vi "getReadStatus.vi"(8 "error in (no error)":errorcluster, 11 "IReaderStatus in":refnum<class "IReaderStatus.lvclass">) -> (0 "error out":errorcluster, 2 "ReadStatus":T1 items=["Ok"=0, "Event"=1, "Fail"=2, "Unknown"=65535], 3 "IReaderStatus out":refnum<class "IReaderStatus.lvclass">)   [LabVIEW 2022 SP3, in "openDAQ.lvlib" / "IBaseObject.lvlib" / "IReaderStatus.lvlib" / "IReaderStatus.lvclass"]
uses:
  <instrlib>/openDAQ/Public/Classes/IReaderStatus/IReaderStatus.lvclass
  C:/Program Files (x86)/National Instruments/LabVIEW 2022/instr.lib/openDAQ/Public/Classes/IBaseObject/IBaseObject.lvclass
  <instrlib>/openDAQ/Public/TypeDef/ReadStatus.ctl
  <instrlib>/openDAQ/Public/Classes/IBaseObject/IBaseObject.lvclass/IBaseObject.ctl
  <instrlib>/openDAQ/Public/Classes/IBaseObject/Accessor/Read reference.vi
  <instrlib>/openDAQ/Public/Classes/IBaseObject/Accessor/Write reference.vi
  <instrlib>/openDAQ/Binaries/Windows/x86/copendaq32.dll
  <instrlib>/openDAQ/openDAQ.lvlib
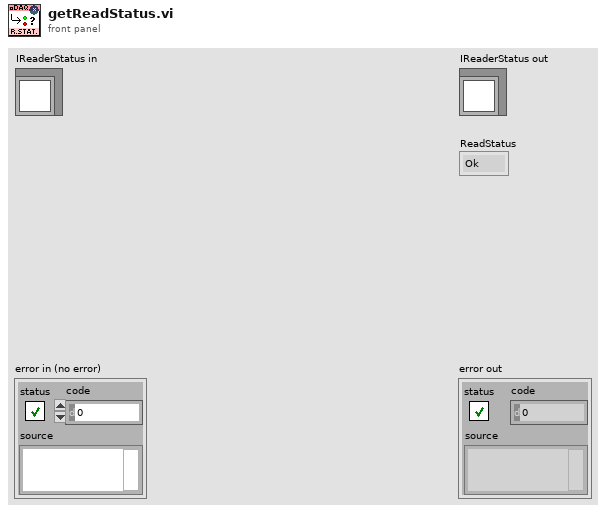
[diagram p1: front panel]
types:
  T1 = typedef "openDAQ.lvlib/ReadStatus.ctl" = u16
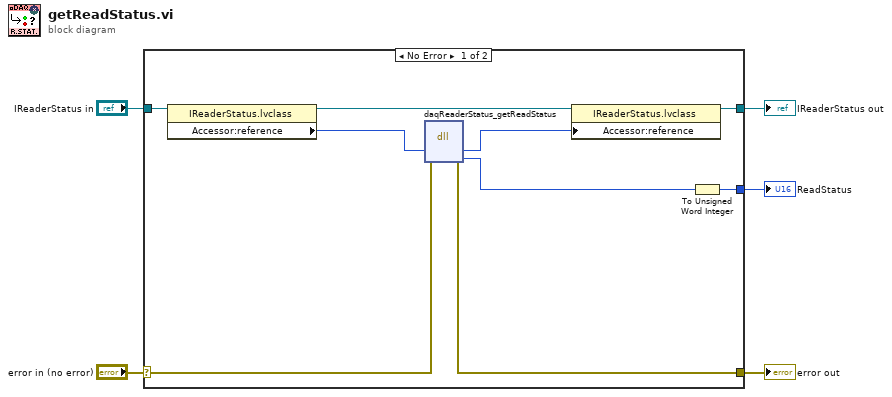
[diagram p0: block diagram]
diagram:
  n1 = case shown="No Error" "error in (no error)" {
    selector: "error in (no error)" -> [w13 w16]
    tunnel: [w12 w16] -> w4
    tunnel: [w10 w15] -> w2
    tunnel: "IReaderStatus in" -> [w14 w15]
    tunnel: [w6 _] -> w1
    frame No Error {
      n2 = property class="IReaderStatus.lvclass"(reference=w14) -> (reference out=w11:refnum<class "IReaderStatus.lvclass">, "Accessor:reference"=w9:i64)  [unwired: 1 in, 1 out]
      n3 = dll-call lib="C:/Program Files (x86)/National Instruments/LabVIEW 2022/instr.lib/openDAQ/Binaries/Windows/x86/copendaq*.*" fn="daqReaderStatus_getReadStatus"(error in=w13, "readerStatus"=w9) -> (error out=w12:errorcluster, "readerStatus"=w8:i64, "status"=w7:i64)  [unwired: 4 in, 1 out]
      n4 = property class="IReaderStatus.lvclass"(reference=w11, "Accessor:reference"=w8) -> (reference out=w10:refnum<class "IReaderStatus.lvclass">)  [unwired: 1 in, 1 out]
      n5 = To Unsigned Word Integer(number=w7) -> (unsigned 16bit integer=w6:u16)
    }
    frame Error {
    }
  }
  "error out" <- w4
  "IReaderStatus out" <- w2
  "ReadStatus" <- w1
